vi "Update.vi"(8 "error in (no error)":errorcluster, 11 "Process in":refnum<class "Process.lvclass">) -> (0 "error out":errorcluster, 3 "Process out":refnum<class "Process.lvclass">)   [LabVIEW 2025, in "Process Actor.lvlib" / "Process.lvclass"]
doc: "This method will cause the actor to send one random number to its caller."
uses:
  Process.lvclass
  <vilib>/ActorFramework/Actor/Actor.lvclass/Actor.ctl
  Process States/Process State Messages/Update from Process Msg/Update from Process Msg.lvclass/Update from Process Msg.ctl
  <vilib>/ActorFramework/Message Enqueuer/Message Enqueuer.lvclass/Message Enqueuer.ctl
  <vilib>/ActorFramework/Message Enqueuer/Enqueue.vi
  Process States/Process State Messages/Update from Process Msg/Update from Process Msg.lvclass
  <vilib>/ActorFramework/Message Priority Queue/Priority Enqueue.vi
  <vilib>/ActorFramework/Actor/Actor.lvclass
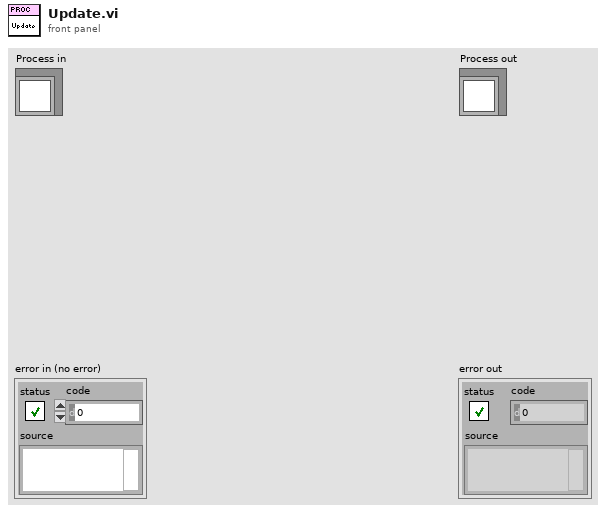
[diagram p1: front panel]
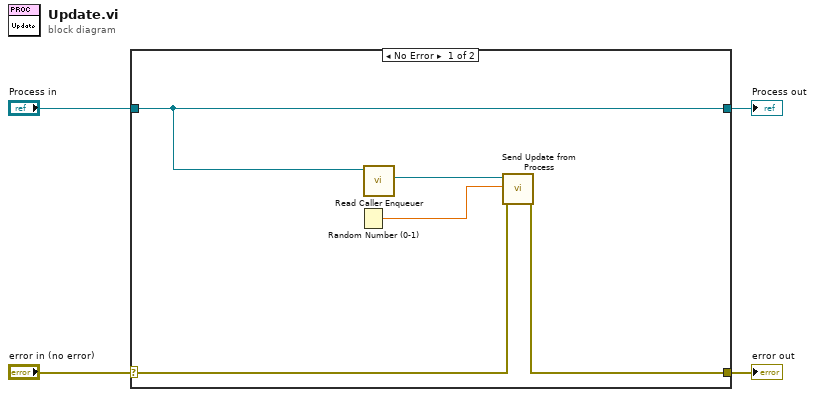
[diagram p0: block diagram]
diagram:
  n1 = case shown="No Error" "error in (no error)" {
    selector: "error in (no error)" -> [w9 w11]
    tunnel: [w8 w11] -> w3
    tunnel: [w7 w10] -> w1
    tunnel: "Process in" -> [w7 w10]
    frame No Error {
      n2 = Random Number (0-1)() -> (number: 0 to 1=w6:dbl)
      n3 = call <vilib>:"Read Caller Enqueuer.vi"("Actor"=w7) -> ("Caller Enqueuer"=w5:refnum<class "Message Enqueuer.lvclass">)  [unwired: 10 in]
      n4 = call "Send Update from Process.vi"("error in (no error)"=w9, "Value"=w6, "Message Enqueuer"=w5) -> ("error out"=w8:errorcluster)  [unwired: 7 in, 1 out]
    }
    frame Error {
    }
  }
  "error out" <- w3
  "Process out" <- w1
